vi "Create New Test Case.vi"(8 "error in (no error)":errorcluster) -> (0 "error out":errorcluster)   [LabVIEW 2020, in "New Test Case.lvlib"]
uses:
  New Test Case.lvlib
  <vilib>/Utility/sysdir.llb/System Directory Type.ctl
  <vilib>/Utility/error.llb/Error Cluster From Error Code.vi
  <vilib>/ErrorRing/Error Ring.xnode
panel:
  in  "Debug?":bool
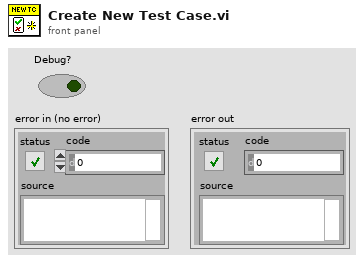
[diagram p1: front panel]
types:
  T1 = enum32{"Invalid", "Standard", "Closed", "Hidden", "Minimized", "Maximized"}
  T2 = typedef "System Directory Type.ctl" = i32
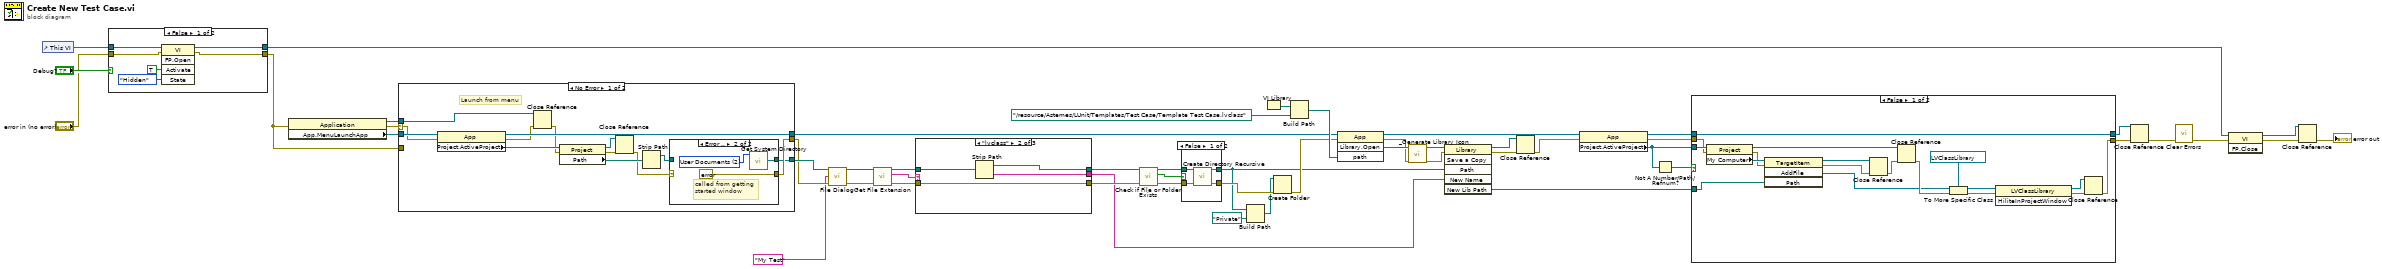
[diagram p0: block diagram]
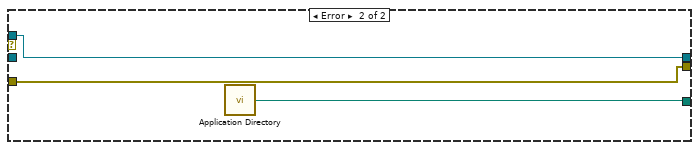
[diagram p3: hidden frame]
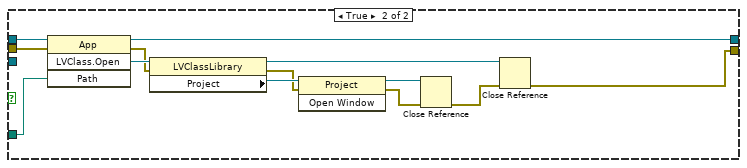
[diagram p5: hidden frame]
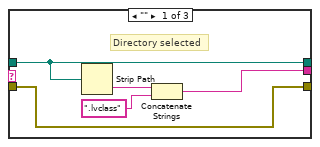
[diagram p6: hidden frame]
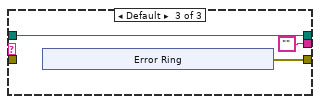
[diagram p7: hidden frame]
diagram:
  n1 = control-ref of="This VI"() -> (w27:refnum<vi>)
  n2 = case shown="False" "Debug?" {
    tunnel: w27 -> [w57 w59]
    tunnel: [w56 w59] -> w25
    tunnel: "error in (no error)" -> [w53 w58]
    tunnel: [w52 w58] -> w17
    frame False {
      n3 = invoke class="VI" method="FP.Open"(reference=w57, error in=w53, "Activate"=TRUE ("Activate?"), "State"=T1."Hidden") -> (reference out=w56:refnum<vi>, error out=w52:errorcluster)  [unwired: 1 in, 3 out]
    }
    frame True {
    }
  }
  n4 = property class="Application"(error in=w17) -> (reference out=w23:refnum<vi>, error out=w29:errorcluster, "App.MenuLaunchApp"=w51:refnum<vi>)  [unwired: 1 in]
  n5 = case shown="No Error" w29 {
    selector: w29 -> [w68 _]
    tunnel: [w71 w81] -> w19
    tunnel: w51 -> [w69 _]
    tunnel: [w62 w80] -> w15
    tunnel: w17 -> [_ w80]
    tunnel: w23 -> [w73 w81]
    tunnel: [w61 w79] -> w16
    frame No Error {
      # "Launch from menu"
      n6 = property class="App"(reference=w69, error in=w68) -> (reference out=w71:refnum<vi>, error out=w70:errorcluster, "Project.ActiveProject"=w72:refnum<vi>)
      n7 = Close Reference(reference=w73, error in (no error)=w70) -> (error out=w67:errorcluster)
      n8 = property class="Project"(reference=w72, error in=w67) -> (reference out=w65:refnum<vi>, error out=w66:errorcluster, "Path"=w64:path)
      n9 = Close Reference(reference=w65, error in (no error)=w66) -> (error out=w63:errorcluster)
      n10 = Strip Path(path=w64) -> (stripped path=w60:path)  [unwired: 1 out]
      n11 = case shown="Error .." w63 {
        selector: w63 -> [w75 _]
        tunnel: [w75 errorcluster {"status"=FALSE, "code"=0, "source"=""} ("error IO")] -> w62
        tunnel: [w74 w76] -> w61
        tunnel: w60 -> [w74 _]
        frame No Error {
        }
        frame Error {
          w77 = T2 2 items=["User Home"=0, "User Desktop"=1, "User Documents"=2, "User Application Data"=3, "User Preferences"=4, "User Temporary"=5, "Public Documents"=6, "Public Application Data"=7, "Public Preferences"=8, "Public Cache"=13, "System Core Libraries"=9, "System Installed Libraries"=10, "Application Files"=11, "Boot Volume Root"=12] ("system directory type")
          # "called from getting started window"
          n12 = call <vilib>:"Get System Directory.vi"("system directory type"=w77) -> ("system directory"=w76:path)  [unwired: 10 in]
        }
      }
    }
    frame Error {
      n13 = call <vilib>:"Application Directory.vi"() -> ("Application Directory"=w79:path)
    }
  }
  n14 = call "File Dialog"("start path"=w16, "default name"="My Test", "error in"=w15) -> ("selected path"=w47:path, "error out"=w14:errorcluster)  [unwired: 9 in, 2 out]
  n15 = call <vilib>:"Get File Extension.vi"("error in (no error)"=w14, "file"=w47) -> ("error out"=w50:errorcluster, "lowercase file extension"=w49:string, "dup file"=w48:path)  [unwired: 5 in, 2 out]
  n16 = case shown="\"lvclass\"" w49 {
    tunnel: w50 -> [w82 w87 _]
    tunnel: w48 -> [w83 w90 w91]
    tunnel: [w82 w87 w93] -> w45
    tunnel: [w84 w89 "" ("name")] -> w41
    tunnel: [w83 w88 w91] -> w46
    frame "" {
      # "Directory selected"
      n17 = Strip Path(path=w83) -> (name=w86:string)  [unwired: 1 out]
      n18 = Concatenate Strings(w86, ".lvclass" ("string")) -> (w84:string)
    }
    frame "lvclass" {
      n19 = Strip Path(path=w90) -> (stripped path=w88:path, name=w89:string)
    }
    frame Default {
      n20 = xnode "Error Ring"() -> ("error out"=w93:errorcluster)
    }
  }
  n21 = call <vilib>:"Check if File or Folder Exists.vi"("error in (no error)"=w45, "path"=w46) -> ("error out"=w44:errorcluster, "file or folder exists?"=w42:bool, "dup path"=w43:path)  [unwired: 7 in]
  n22 = case shown="False" w42 {
    tunnel: w44 -> [w101 w102]
    tunnel: w43 -> [w100 w103]
    tunnel: [w99 w103] -> w10
    tunnel: [w98 w102] -> w13
    frame False {
      n23 = call <vilib>:"Create Directory Recursive.vi"("error in (no error)"=w101, "directory"=w100) -> ("error out"=w98:errorcluster, "directory copy"=w99:path)  [unwired: 3 in, 1 out]
    }
    frame True {
    }
  }
  n24 = Build Path(base path=w10, name or relative path=path "Private") -> (appended path=w8:path)
  n25 = VI Library() -> (path=w34:path)
  n26 = Create Folder(path (use dialog)=w8, error in=w13) -> (error out=w11:errorcluster)  [unwired: 1 in, 2 out]
  n27 = Build Path(base path=w34, name or relative path=path "../resource/Astemes/LUnit/Templates/Test Case/Template Test Case.lvclass") -> (appended path=w32:path)
  n28 = invoke class="App" method="Library.Open"(reference=w19, error in=w11, "path"=w32) -> (reference out=w5:refnum<vi>, error out=w1:errorcluster, "Open Library"=w4:refnum<vi>)  [unwired: 1 in, 1 out]
  n29 = call "_Generate Library Icon.vi"("error in (no error)"=w1, "Library"=w4) -> ("error out"=w2:errorcluster, "Library out"=w3:refnum<vi>)  [unwired: 8 in]
  n30 = invoke class="Library" method="Save a Copy"(reference=w3, error in=w2, "Path"=w10, "New Name"=w41) -> (reference out=w30:refnum<vi>, error out=w28:errorcluster, "New Lib Path"=w7:path)  [unwired: 2 in, 3 out]
  n31 = Close Reference(reference=w30, error in (no error)=w28) -> (error out=w6:errorcluster)
  n32 = property class="App"(reference=w5, error in=w6) -> (reference out=w37:refnum<vi>, error out=w38:errorcluster, "Project.ActiveProject"=w39:refnum<vi>)
  n33 = Not A Number/Path/Refnum?(number/path/refnum=w39) -> (NaN/Path/Refnum?=w40:bool)
  n34 = case shown="False" w40 {
    tunnel: w39 -> [w121 _]
    tunnel: w38 -> [w119 w125]
    tunnel: w7 -> [w113 w123]
    tunnel: [w108 w122] -> w35
    tunnel: w37 -> [w112 w126]
    tunnel: [w112 w124] -> w36
    frame False {
      n35 = property class="Project"(reference=w121, error in=w119) -> (reference out=w115:refnum<vi>, error out=w118:errorcluster, "My Computer"=w120:refnum<vi>)
      n36 = invoke class="TargetItem" method="AddFile"(reference=w120, error in=w118, "Path"=w113) -> (reference out=w116:refnum<vi>, error out=w117:errorcluster, "AddFile"=w104:refnum<vi>)  [unwired: 1 in, 1 out]
      n37 = Close Reference(reference=w116, error in (no error)=w117) -> (error out=w114:errorcluster)
      n38 = Close Reference(reference=w115, error in (no error)=w114) -> (error out=w111:errorcluster)
      n39 = To More Specific Class(target class=refnum<vi> refnum ("reference"), reference=w104, error in=w111) -> (specific class reference=w105:refnum<vi>, error out=w107:errorcluster)
      n40 = invoke class="LVClassLibrary" method="HiliteInProjectWindow"(reference=w105, error in=w107) -> (reference out=w109:refnum<vi>, error out=w110:errorcluster)  [unwired: 1 in, 1 out]
      n41 = Close Reference(reference=w109, error in (no error)=w110) -> (error out=w108:errorcluster)
    }
    frame True {
      n42 = invoke class="App" method="LVClass.Open"(reference=w126, error in=w125, "Path"=w123) -> (reference out=w124:refnum<vi>, error out=w133:errorcluster, "LVClass.Open"=w134:refnum<vi>)  [unwired: 1 in, 1 out]
      n43 = property class="LVClassLibrary"(reference=w134, error in=w133) -> (reference out=w132:refnum<vi>, error out=w130:errorcluster, "Project"=w131:refnum<vi>)
      n44 = invoke class="Project" method="Open Window"(reference=w131, error in=w130) -> (reference out=w129:refnum<vi>, error out=w128:errorcluster)  [unwired: 1 in, 1 out]
      n45 = Close Reference(reference=w129, error in (no error)=w128) -> (error out=w127:errorcluster)
      n46 = Close Reference(reference=w132, error in (no error)=w127) -> (error out=w122:errorcluster)
    }
  }
  n47 = Close Reference(reference=w36, error in (no error)=w35) -> (error out=w31:errorcluster)
  n48 = call <vilib>:"Clear Errors.vi"("error in (no error)"=w31) -> ("error out"=w20:errorcluster)  [unwired: 5 in, 1 out]
  n49 = invoke class="VI" method="FP.Close"(reference=w25, error in=w20) -> (reference out=w22:refnum<vi>, error out=w21:errorcluster)  [unwired: 1 in, 1 out]
  n50 = Close Reference(reference=w22, error in (no error)=w21) -> (error out=→"error out":errorcluster)
